vi "Send Read Parameters.vi"(7 "Message Priority (Normal)":T1=enum."Normal", 8 "error in (no error)":errorcluster, 9 "timeout in ms (-1)":i32=-1, 11 "Message Enqueuer":refnum<class "Message Enqueuer.lvclass">) -> (0 "error out":errorcluster, 1 "timed out?":bool, 2 "Parameters":refnum<class "Mag Lab Parameters.lvclass">, 3 "Message Enqueuer out":refnum<class "Message Enqueuer.lvclass">)   [LabVIEW 2015, in "Read Parameters Msg.lvclass"]
doc: "This VI sends the message to an actor."
uses:
  Read Parameters Msg.lvclass
  <vilib>/ActorFramework/Message Enqueuer/Message Enqueuer.lvclass
  <vilib>/ActorFramework/Message Enqueuer/Message Priority.ctl
  Mag Lab Properties/Mag Lab Parameters.lvclass
  <vilib>/ActorFramework/Reply Msg/Reply Msg.lvclass/Reply Msg.ctl
  <vilib>/ActorFramework/Message Enqueuer/Message Enqueuer.lvclass/Message Enqueuer.ctl
  <vilib>/ActorFramework/Message Enqueuer/Enqueue.vi
  <vilib>/ActorFramework/Message Priority Queue/Priority Enqueue.vi
  <vilib>/ActorFramework/Reply Msg/Reply Msg.lvclass
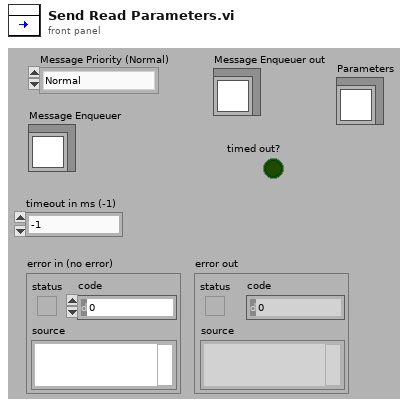
[diagram p1: front panel]
types:
  T1 = typedef "Actor Framework.lvlib/Message Enqueuer.lvclass/Message Priority.ctl" = enum16{"Low", "Normal", "High"}
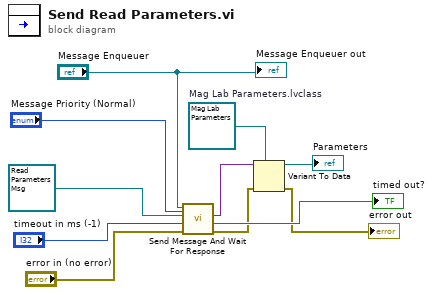
[diagram p0: block diagram]
diagram:
  w6 = refnum<class "Mag Lab Parameters.lvclass"> refnum  # Mag Lab Parameters.lvclass
  n1 = call <vilib>:"Send Message And Wait For Response.vi"("Message Priority (Normal)"="Message Priority (Normal)", "error in (no error)"="error in (no error)", "timeout in ms (-1)"="timeout in ms (-1)", "Original Message"=refnum<class "Read Parameters Msg.lvclass"> refnum ("Object"), "Message Enqueuer in"="Message Enqueuer") -> ("error out"=w4:errorcluster, "timed out?"=→"timed out?":bool, "Reply"=w7:variant)  [unwired: 3 in, 1 out]
  n2 = Variant To Data(error in=w4, type=w6, Variant=w7) -> (data=→"Parameters":refnum<class "Mag Lab Parameters.lvclass">, error out=→"error out":errorcluster)
  "Message Enqueuer out" <- "Message Enqueuer"
